vi "Stage Resolution Test_YCC.vi"() -> ()   [LabVIEW 2014]
uses:
  (Global) Current handle and LaserPower_YCC.vi
panel:
  out "Cal R.S (nm)":dbl
  out "mean now precise position (nm) 2":dbl format="%0.5f"
  out "mean now precise position (nm)":dbl format="%0.5f"
  in  "R.S. test (nm)":dbl=1.0
  in  "axis":u32=1
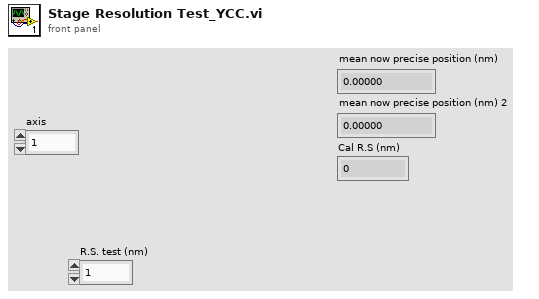
[diagram p1: front panel]
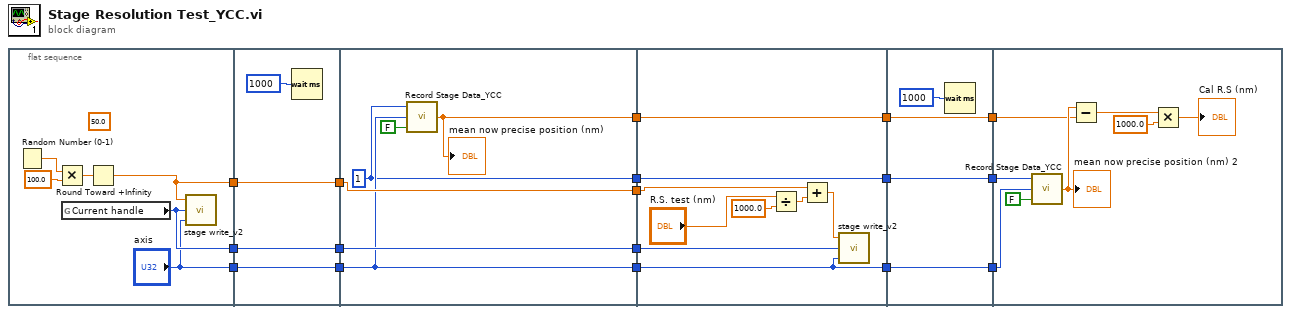
[diagram p0: block diagram]
diagram:
  n1 = flat-sequence {
    tunnel: [w18] -> w12
    tunnel: [w23] -> w10
    tunnel: ["axis"] -> w8
    tunnel: w12 -> [w27]
    tunnel: [w27] -> w11
    tunnel: w10 -> [w26]
    tunnel: [w26] -> w9
    tunnel: w8 -> [w25]
    tunnel: [w25] -> w7
    tunnel: w11 -> [w33]
    tunnel: [w33] -> w17
    tunnel: w9 -> [w32]
    tunnel: [w32] -> w16
    tunnel: w7 -> [w31]
    tunnel: [w31] -> w15
    tunnel: [w30] -> w14
    tunnel: [w28] -> w13
    tunnel: w17 -> [w39]
    tunnel: w16 -> [w37]
    tunnel: w15 -> [w36]
    tunnel: [w36] -> w6
    tunnel: [w35] -> w4
    tunnel: w14 -> [w35]
    tunnel: [w34] -> w2
    tunnel: w13 -> [w34]
    tunnel: w6 -> [w46]
    tunnel: [w46] -> w5
    tunnel: w4 -> [w45]
    tunnel: [w45] -> w3
    tunnel: w2 -> [w44]
    tunnel: [w44] -> w1
    tunnel: w5 -> [w54]
    tunnel: w3 -> [w52]
    tunnel: w1 -> [w47]
    frame #0 {
      (unwired) 50.0 ("position")
      n2 = Random Number (0-1)() -> (number: 0 to 1=w21:dbl)
      n3 = Multiply(x=w21, y=100.0) -> (x*y=w19:dbl)
      n4 = global read "(Global) Current handle and LaserPower_YCC.vi" "Current handle"() -> (w23:i32)
      n5 = Round Toward +Infinity(x=w19) -> (ceil(x): smallest int >= x=w18:dbl)
      n6 = call "stage write_v2.vi"("axis"="axis", "Incoming Handle"=w23, "position"=w18) -> ()  [unwired: 2 in, 1 out]
    }
    frame #1 {
      n7 = Wait (ms)(milliseconds to wait=u32 1000) -> ()  [unwired: 1 out]
    }
    frame #2 {
      w28 = u32 1 ("Record time (s)")
      n8 = call "Record Stage Data_YCC.vi"("Save Data?"=FALSE, "Axis"=w31, "Record time (s)"=w28) -> ("mean now precise position (nm)"=w30:dbl)  [unwired: 1 in, 1 out]
      "mean now precise position (nm)" <- w30
    }
    frame #3 {
      n9 = Divide(x="R.S. test (nm)", y=1000.0 ("position")) -> (x/y=w40:dbl)
      n10 = Add(x=w39, y=w40) -> (x+y=w38:dbl)
      n11 = call "stage write_v2.vi"("axis"=w36, "Incoming Handle"=w37, "position"=w38) -> ()  [unwired: 2 in, 1 out]
    }
    frame #4 {
      n12 = Wait (ms)(milliseconds to wait=u32 1000) -> ()  [unwired: 1 out]
    }
    frame #5 {
      n13 = call "Record Stage Data_YCC.vi"("Save Data?"=FALSE, "Axis"=w54, "Record time (s)"=w47) -> ("mean now precise position (nm)"=w53:dbl)  [unwired: 1 in, 1 out]
      "mean now precise position (nm) 2" <- w53
      n14 = Subtract(x=w53, y=w52) -> (x-y=w51:dbl)
      n15 = Multiply(x=w51, y=1000.0 ("position")) -> (x*y=→"Cal R.S (nm)":dbl)
    }
  }
